vi "serialDriver.vi"(6 "Serial Port Enum":T1, 8 "Error In":errorcluster, 10 "Value In":string, 11 "VISA resource name":refnum<visa-resource-name>) -> (0 "Error Out":errorcluster, 3 "Value Out":string)   [LabVIEW 2018]
uses:
  controls/serialPortEnum.ctl
  <vilib>/Instr/_visa.llb/VISA Configure Serial Port (Instr).vi
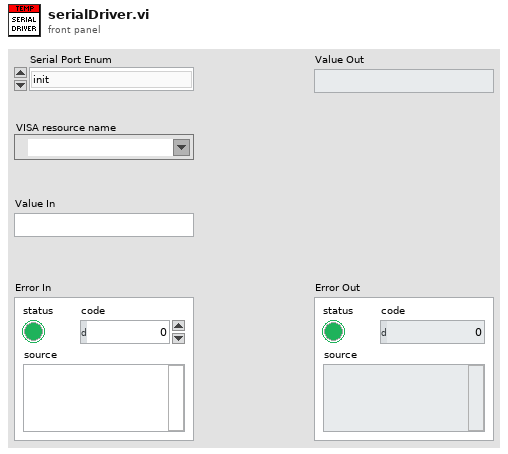
[diagram p1: front panel]
types:
  T1 = typedef "serialPortEnum.ctl" = enum16{"init", "write", "read", "close"}
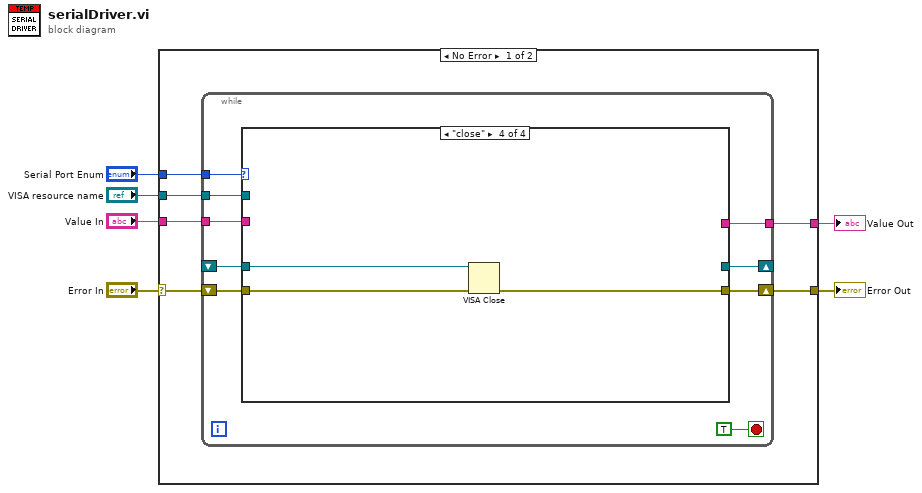
[diagram p0: block diagram]
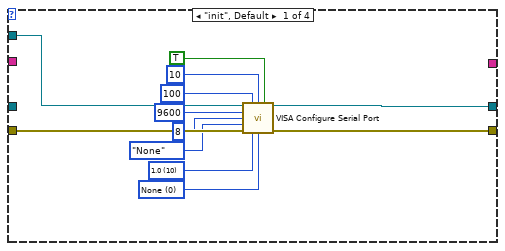
[diagram p2: hidden frame]
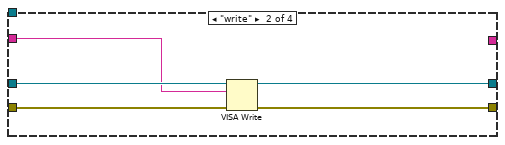
[diagram p3: hidden frame]
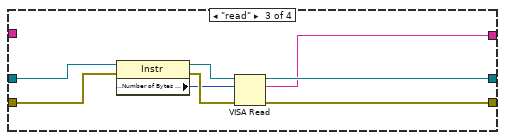
[diagram p4: hidden frame]
diagram:
  n1 = case shown="No Error" "Error In" {
    selector: "Error In" -> [w12 w50]
    tunnel: [w11 w50] -> w3
    tunnel: "Serial Port Enum" -> [w10 _]
    tunnel: "VISA resource name" -> [w9 _]
    tunnel: "Value In" -> [w8 _]
    tunnel: [w7 _] -> w1
    frame No Error {
      n2 = while {
        tunnel: w10 -> [w19]
        shift-right: [w20] -> w11
        shift-left: w12 -> [w21]
        shift-right: [w18] -> _
        shift-left: _ -> [w17]
        tunnel: w9 -> [w15]
        tunnel: w8 -> [w14]
        tunnel: [w13] -> w7
        stop <- TRUE stop-if-true
        n3 = case shown="\"close\"" w19 {
          tunnel: w21 -> [w32 w37 w43 w47]
          tunnel: [w33 w38 w45 w49] -> w20
          tunnel: [w31 w36 w46 _] -> w18
          tunnel: w17 -> [_ w35 w44 w48]
          tunnel: w15 -> [w30 _ _ _]
          tunnel: w14 -> [_ w34 _ _]
          tunnel: [_ _ w39 _] -> w13
          frame "init", Default {
            w22 = u16 0 items=["None", "XON/XOFF", "RTS/CTS", "XON/XOFF & RTS/CTS", "DTR/DSR", "XON/XOFF & DTR/DSR"] ("flow control (0:none)")
            w23 = u16 10 items=["1.0"=10, "1.5"=15, "2.0"=20] ("stop bits (10: 1 bit)")
            n4 = call-poly "VISA Configure Serial Port"("VISA resource name"=w30, "timeout (10sec)"=u32 100, "termination char\n(0xA = '\\n' = LF)"=u8 10 ("termination char\n(0xA = '\\n' = LF)"), "Enable Termination\nChar (T)"=TRUE ("Enable Termination\nChar (T)"), "baud rate (9600)"=u32 9600, "data bits (8)"=u16 8, "parity (0:none)"=enum16{"None", "Odd", "Even", "Mark", "Space"}."None", "error in (no error)"=w32, "stop bits (10: 1 bit)"=w23, "flow control (0:none)"=w22) -> ("VISA resource name out"=w31:refnum<visa-resource-name>, "error out"=w33:errorcluster)  [unwired: 4 in]
          }
          frame "write" {
            n5 = VISA Write(VISA resource name=w35, write buffer=w34, error in (no error)=w37) -> (VISA resource name out=w36:refnum<visa-resource-name>, error out=w38:errorcluster)  [unwired: 1 out]
          }
          frame "read" {
            n6 = property class="Instr"(reference=w44, error in=w43) -> (reference out=w41:refnum<visa-resource-name>, error out=w42:errorcluster, "Serial Settings:Number of Bytes at Serial Port"=w40:u32)
            n7 = VISA Read(VISA resource name=w41, byte count=w40, error in (no error)=w42) -> (VISA resource name out=w46:refnum<visa-resource-name>, read buffer=w39:string, error out=w45:errorcluster)  [unwired: 1 out]
          }
          frame "close" {
            n8 = VISA Close(VISA resource name=w48, error in (no error)=w47) -> (error out=w49:errorcluster)
          }
        }
      }
    }
    frame Error {
    }
  }
  "Value Out" <- w1
  "Error Out" <- w3
